vi "CloseVISA.vi"(1 "VISA Resource Name":refnum<visa-resource-name>) -> (0 "error out":errorcluster)   [LabVIEW 2010]
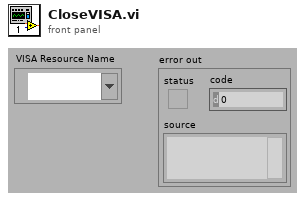
[diagram p1: front panel]
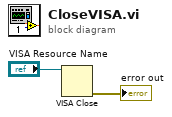
[diagram p0: block diagram]
diagram:
  n1 = VISA Close(VISA resource name="VISA Resource Name") -> (error out=→"error out":errorcluster)  [unwired: 1 in]
